vi "push.vi"(9 "Push":dbl, 10 "Before":dbl[](array[numeric])) -> (2 "After":dbl[](array[numeric]))   [LabVIEW 2009]
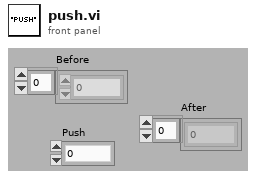
[diagram p1: front panel]
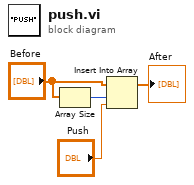
[diagram p0: block diagram]
diagram:
  n1 = Array Size(array="Before") -> (size(s)=w1:i32)
  n2 = Insert Into Array(array="Before", index=w1, new element="Push") -> (→"After":dbl[])
